vi "Clear_Lines.vi"(11 "Retain?":bool) -> ()   [LabVIEW 2019]
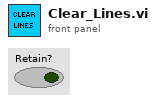
[diagram p1: front panel]
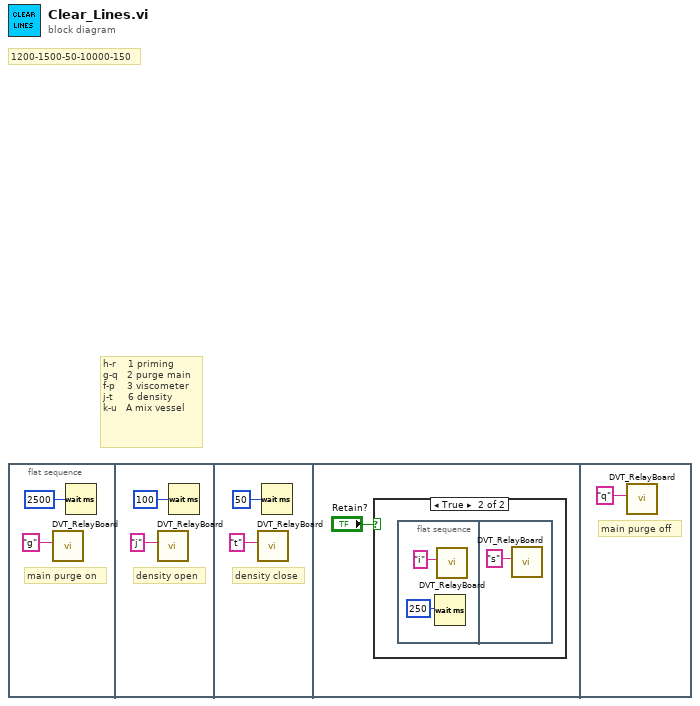
[diagram p0: block diagram]
diagram:
  # "1200-1500-50-10000-150"
  # "h-r    1 priming\ng-q   2 purge main\nf-p    3 viscometer\nj-t     6 density\nk-u   A mix vessel"
  n1 = flat-sequence {
    frame #0 {
      # "main purge on"
      n2 = call "DVT_RelayBoard.vi"("write buffer"="g") -> ()  [unwired: 3 in, 3 out]
      n3 = Wait (ms)(milliseconds to wait=u32 2500) -> ()  [unwired: 1 out]
    }
    frame #1 {
      # "density open"
      n4 = call "DVT_RelayBoard.vi"("write buffer"="j") -> ()  [unwired: 3 in, 3 out]
      n5 = Wait (ms)(milliseconds to wait=u32 100) -> ()  [unwired: 1 out]
    }
    frame #2 {
      # "density close"
      n6 = call "DVT_RelayBoard.vi"("write buffer"="t") -> ()  [unwired: 3 in, 3 out]
      n7 = Wait (ms)(milliseconds to wait=u32 50) -> ()  [unwired: 1 out]
    }
    frame #3 {
      n8 = case shown="True" "Retain?" {
        frame False {
        }
        frame True {
          n9 = flat-sequence {
            frame #0 {
              n10 = Wait (ms)(milliseconds to wait=u32 250) -> ()  [unwired: 1 out]
              n11 = call "DVT_RelayBoard.vi"("write buffer"="i") -> ()  [unwired: 3 in, 3 out]
            }
            frame #1 {
              n12 = call "DVT_RelayBoard.vi"("write buffer"="s") -> ()  [unwired: 3 in, 3 out]
            }
          }
        }
      }
    }
    frame #4 {
      # "main purge off"
      n13 = call "DVT_RelayBoard.vi"("write buffer"="q") -> ()  [unwired: 3 in, 3 out]
    }
  }
